vi "VXM Com.vi"(4 "Flush RS232":bool, 6 "Timeout, s":dbl=0.25, 7 "Operation":T1(ring), 8 "error in (no error)":errorcluster, 9 "Termination String ('/' codes)":string, 10 "Write Buffer ('/' codes)":string, 11 "VISA resource name":refnum<visa-resource-name>) -> (0 "error out":errorcluster, 2 "Response String ('/' codes)":string, 3 "VISA resource out":refnum<visa-resource-name>)   [LabVIEW 2017]
doc: "Low-level communicator VI for Velmex VXM controller.\nAll-in-one, has a lot of different configurations.\nPuts all comm into one, central location."
panel:
  out "debug":string[](array[string])
  out "i":i32
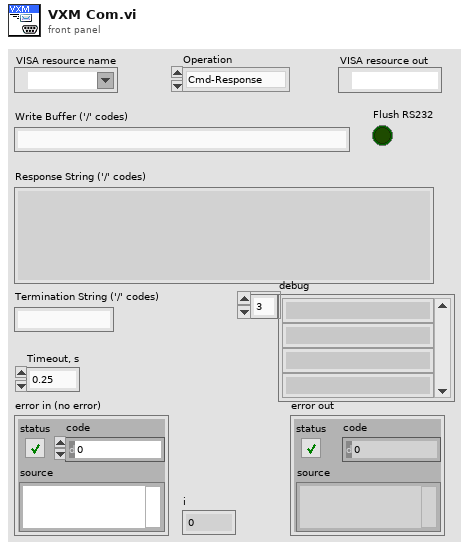
[diagram p1: front panel]
types:
  T1 = enum16{"Cmd-Response", "Write Only", "Read Only"}
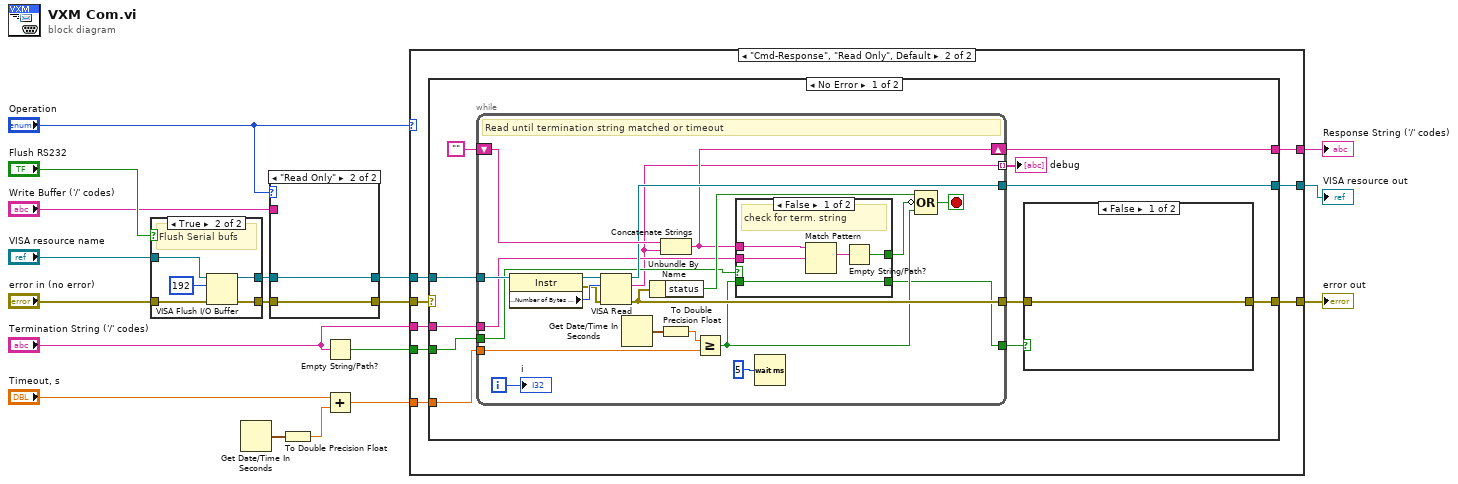
[diagram p0: block diagram]
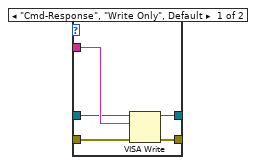
[diagram p3: hidden frame]
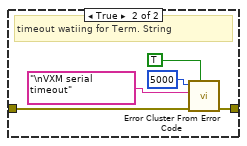
[diagram p5: hidden frame]
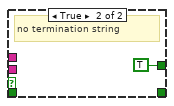
[diagram p6: hidden frame]
diagram:
  n1 = case shown="True" "Flush RS232" {
    tunnel: [w19 w25] -> w6
    tunnel: "error in (no error)" -> [w19 w24]
    tunnel: "VISA resource name" -> [w20 w22]
    tunnel: [w20 w21] -> w1
    frame False {
    }
    frame True {
      # "Flush Serial bufs"
      n2 = VISA Flush I/O Buffer(VISA resource name=w22, mask (16)=u16 192, error in (no error)=w24) -> (VISA resource name out=w21:refnum<visa-resource-name>, error out=w25:errorcluster)
    }
  }
  n3 = Get Date/Time In Seconds() -> (seconds since 1Jan1904=w18:timestamp)
  n4 = case shown="\"Read Only\"" "Operation" {
    tunnel: [w30 w31] -> w14
    tunnel: w6 -> [w27 w32]
    tunnel: [w29 w32] -> w10
    tunnel: "Write Buffer ('/' codes)" -> [w28 _]
    tunnel: w1 -> [w26 w31]
    frame "Cmd-Response", "Write Only", Default {
      # "Write VISA string to instrument"
      n5 = VISA Write(VISA resource name=w26, write buffer=w28, error in (no error)=w27) -> (VISA resource name out=w30:refnum<visa-resource-name>, error out=w29:errorcluster)  [unwired: 1 out]
    }
    frame "Read Only" {
      # "Read only, don't write"
    }
  }
  n6 = To Double Precision Float(number=w18) -> (double precision float=w17:dbl)
  n7 = Empty String/Path?(string/path="Termination String ('/' codes)") -> (empty?=w8:bool)
  n8 = Add(x="Timeout, s", y=w17) -> (x+y=w15:dbl)
  n9 = case shown="\"Cmd-Response\", \"Read Only\", Default" "Operation" {
    tunnel: w15 -> [_ w42]
    tunnel: w14 -> [w34 w41]
    tunnel: [_ w40] -> w13
    tunnel: [w34 w39] -> w12
    tunnel: [w33 w38] -> w11
    tunnel: w10 -> [w33 w37]
    tunnel: "Termination String ('/' codes)" -> [_ w36]
    tunnel: w8 -> [_ w35]
    frame "Write Only" {
      # "Write only"
    }
    frame "Cmd-Response", "Read Only", Default {
      # "Query = read bytes back"
      n10 = case shown="No Error" w37 {
        selector: w37 -> [_ w88]
        tunnel: w42 -> [w53 _]
        tunnel: w41 -> [w51 w87]
        tunnel: [w50 _] -> w40
        tunnel: w36 -> [w49 _]
        tunnel: [w47 w87] -> w39
        tunnel: [w46 w88] -> w38
        tunnel: w35 -> [w44 _]
        frame No Error {
          n11 = while {
            tunnel: w53 -> [w63]
            shift-right: [w61] -> w50
            shift-left: "" -> [w75]
            tunnel: [w74] -> w47
            tunnel: w51 -> [w73]
            tunnel: w49 -> [w70]
            tunnel: [w64] -> w48
            tunnel: [w68] -> w45
            tunnel: w44 -> [w67]
            tunnel: [w60] -> w43 mode=indexing
            i -> [w66]
            stop <- w69 stop-if-true
            # "Read until termination string matched or timeout"
            n12 = property class="Instr"(reference=w73) -> (reference out=w76:refnum<visa-resource-name>, error out=w77:errorcluster, "Serial Settings:Number of Bytes at Serial Port"=w78:u32)  [unwired: 1 in]
            n13 = VISA Read(VISA resource name=w76, byte count=w78, error in (no error)=w77) -> (VISA resource name out=w74:refnum<visa-resource-name>, read buffer=w60:string, error out=w68:errorcluster)  [unwired: 1 out]
            n14 = Get Date/Time In Seconds() -> (seconds since 1Jan1904=w80:timestamp)
            n15 = Unbundle By Name(w68) -> ("status"=w71:bool)
            n16 = Concatenate Strings(w75, w60) -> (w61:string)
            n17 = To Double Precision Float(number=w80) -> (double precision float=w62:dbl)
            n18 = Greater Or Equal?(x=w62, y=w63) -> (x >= y?=w65:bool)
            n19 = case shown="False" w67 {
              tunnel: [w85 TRUE] -> w72
              tunnel: w61 -> [w83 _]
              tunnel: w70 -> [w82 _]
              tunnel: [w81 _] -> w64
              tunnel: w65 -> [w81 _]
              frame False {
                # "check for term. string"
                n20 = Match Pattern(string=w83, regular expression=w82) -> (match substring=w84:string)  [unwired: 1 in, 3 out]
                n21 = Empty String/Path?(string/path=w84) -> (empty?=w85:bool)
              }
              frame True {
                # "no termination string"
              }
            }
            n22 = Wait (ms)(milliseconds to wait=u32 5) -> ()  [unwired: 1 out]
            n23 = Compound Arithmetic op=OR(w71, invert w72, w65) -> (w69:bool)
            "i" <- w66
          }
          "debug" <- w43
          n24 = case shown="False" w48 {
            tunnel: [w54 w56] -> w46
            tunnel: w45 -> [w54 w55]
            frame False {
            }
            frame True {
              # "timeout watiing for Term. String"
              n25 = call <vilib>:"Error Cluster From Error Code.vi"("show call chain? (False)"=TRUE, "error in (no error)"=w55, "error message (\"\")"="\nVXM serial timeout" ("ErrorDescription"), "error code (0)"=5000 ("ErrorCode")) -> ("error out"=w56:errorcluster)  [unwired: 5 in]
            }
          }
        }
        frame Error {
        }
      }
    }
  }
  "Response String ('/' codes)" <- w13
  "error out" <- w11
  "VISA resource out" <- w12
